vi "crio_RT_Antagonist_Axial_Sine_Sweep.vi"() -> ()   [LabVIEW 2019]
uses:
  <vilib>/LabVIEW Targets/FPGA/cRIO/shared/nicrio_ModuleControls/nicrio_cRIO-9237_ExcitationVoltageRing.ctl
  <vilib>/Platform/TimedLoop/XDataNode/timing_clust.ctl
  <vilib>/Platform/TimedLoop/XDataNode/nitl_modes.ctl
  <vilib>/Platform/TimedLoop/XDataNode/wakeup.ctl
  <vilib>/FPGAPlugInAG/cRIO-9074/niLvFpga_Open_cRIO-9074.vi
  <vilib>/rvi/interface/common/dynamic/niFpgaDynamicAddResources.vi
  <vilib>/Utility/error.llb/Error Cluster From Error Code.vi
  <vilib>/rvi/errors/niLvFpgaAdjustHostInterfaceError.vi
  <vilib>/FPGAPlugInAG/Dynamic/niLvFpga_Close_Dynamic.vi
  <vilib>/rvi/interface/nirviOpenFPGA/nirviOpenFPGA.xnode
  On Call Bitfiles/gpass2_FPGATarget2_crioFPGAAntagoni_YEb8loNiaqg.lvbitx
  <vilib>/rvi/interface/nirviReadWriteControl/nirviReadWriteControl.xnode
  <vilib>/platform/TimedLoop/XDataNode/XDataNode.xnode
  <vilib>/rvi/interface/nirviCloseFPGA/nirviCloseFPGA.xnode
  NiFpgaLv.dll
  <vilib>/rvi/interface/Simulation/niFpgaSimulationCallBeginRW.vi
  <vilib>/Platform/TimedLoop/XDataNode/XDNodeRunTimeDep.lvlib
panel:
  out "PWM":sgl(graph)=0.061072454
  out "Load Cell":dbl(graph)
  in  "LAC Gains":T1={"proportional gain"=0.95454544, "integral gain"=0.64646465} {"proportional gain" scale=0.0..1.0; "integral gain" scale=0.0..1.0}
  in  "LAC Gain Scaler":T1={"proportional gain"=100.0, "integral gain"=100000000.0}
  in  "LAC manual control":T2={"manual? (F)"=FALSE, "manual input (0)"=-0.83838385} {"manual input (0)" scale=-1.0..1.0}
  out "LAC Measured Position":i32
  in  "LAC setpoint":i32(slide) scale=0.0..4500.0
  out "LAC Actual Gain":T1={"proportional gain"=0.009545455, "integral gain"=1.2626262e-09}
  in  "Excitation Voltage":T3 items=["2.5 Volts", "3.3 Volts", "5.0 Volts", "10.0 Volts", "External Excitation"]
  out "Position (Counts) VCA":i32=1
  in  "Lock_debug":bool
  in  "Idle Frequency":dbl=1.0
  in  "Lock_loop_rate":u32=5000
  out "magnitude":fxp<+,32,6>=14.0474853515625
  out "phase (pi)":fxp<+/-,16,2>=0.27923583984375
  out "lock_input":fxp<+/-,16,5>=2.0
  in  "sin_gain":fxp<+,16,2>
  in  "sin_offset":fxp<+/-,16,3>
  out "ControllerPWM Output":sgl=0.5
  out "Mod1/AI0":fxp<+/-,24,-4>=2.2202730178833008e-06
  out "scaled load cell reading":fxp<+/-,24,24>=2.0
  out "Phase":dbl(graph)=-15.1611328125
  out "Phase Graph":cluster{dbl, dbl}[](graph)=[{0.2, -26.400146484375}, {0.25, -26.400146484375}, {0.30000000000000004, -26.982421875}, {0.35000000000000003, -27.70751953125}, {0.4, -27.70751953125}, {0.45, -27.70751953125}, {0.5, -28.80615234375}, {0.55, -28.80615234375}, {0.6000000000000001, -28.80615234375}, {0.65, -29.937744140625}, {0.7, -30.311279296875}, {0.75, -30.311279296875}, {0.8, -31.39892578125}, {0.8500000000000001, -31.915283203125}, {0.9000000000000001, -31.915283203125}, {0.95, -31.915283203125}, {1.0, -32.222900390625}, {1.05, -32.7392578125}, {1.1, -32.84912109375}, {1.1500000000000001, -32.84912109375}, {1.2, -32.84912109375}, {1.25, -33.563232421875}, {1.3, -34.2333984375}, {1.35, -34.2333984375}, {1.4000000000000001, -34.595947265625}, {1.45, -34.947509765625}, {1.5, -35.26611328125}, {1.55, -35.804443359375}, {1.6, -35.804443359375}, {1.6500000000000001, -35.947265625}, {1.7, -36.156005859375}, {1.75, -36.551513671875}, {1.8, -36.595458984375}, {1.85, -36.595458984375}, {1.9000000000000001, -36.93603515625}, {1.95, -36.93603515625}, {2.0, -36.93603515625}, {2.0500000000000003, -37.606201171875}, {2.1, -37.606201171875}, {2.1500000000000004, -38.704833984375}, {2.2, -38.704833984375}, {2.2500000000000004, -38.704833984375}, {2.3000000000000003, -39.3310546875}, {2.35, -39.3310546875}, {2.4000000000000004, -39.3310546875}, {2.45, -40.18798828125}, {2.5000000000000004, -40.18798828125}, {2.5500000000000003, -40.18798828125}, {2.6000000000000005, -41.033935546875}, {2.6500000000000004, -41.033935546875}, {2.7, -41.6162109375}, {2.7500000000000004, -41.6162109375}, {2.8000000000000003, -41.6162109375}, {2.8500000000000005, -42.451171875}, {2.9000000000000004, -42.451171875}, {2.95, -42.91259765625}, {3.0000000000000004, -42.91259765625}, {3.0500000000000003, -42.91259765625}, {3.1000000000000005, -42.91259765625}, {3.1500000000000004, -43.9013671875}, {3.2, -44.9560546875}, {3.2500000000000004, -44.9560546875}, {3.3000000000000003, -44.9560546875}, {3.3500000000000005, -45.46142578125}, {3.4000000000000004, -45.46142578125}, {3.45, -46.680908203125}, {3.5000000000000004, -47.63671875}, {3.5500000000000003, -48.3837890625}, {3.6000000000000005, -48.3837890625}, {3.6500000000000004, -49.339599609375}, {3.7, -49.339599609375}, {3.7500000000000004, -50.372314453125}, {3.8000000000000003, -51.48193359375}, {3.8500000000000005, -51.48193359375}, {3.9000000000000004, -52.283935546875}, {3.95, -52.283935546875}, {4.0, -52.283935546875}, {4.05, -54.60205078125}, {4.1000000000000005, -56.44775390625}, {4.15, -56.44775390625}, {4.2, -57.535400390625}, {4.25, -57.535400390625}, {4.300000000000001, -59.69970703125}, {4.3500000000000005, -62.7978515625}, {4.4, -62.7978515625}, {4.45, -62.7978515625}, {4.5, -66.236572265625}, {4.550000000000001, -66.236572265625}, {4.6000000000000005, -66.236572265625}, {4.65, -66.236572265625}, {4.7, -75.574951171875}, {4.75, -75.574951171875}, {4.800000000000001, -77.838134765625}, {4.8500000000000005, -79.013671875}, {4.9, -79.793701171875}, {4.95, -79.793701171875}, {5.000000000000001, -79.793701171875}, {5.050000000000001, -79.793701171875}, {5.1000000000000005, -86.099853515625}, {5.15, -92.30712890625}, {5.2, -92.30712890625}, {5.250000000000001, -95.8447265625}, {5.300000000000001, -95.8447265625}, {5.3500000000000005, -99.173583984375}, {5.4, -103.831787109375}, {5.45, -103.831787109375}, {5.500000000000001, -105.897216796875}, {5.550000000000001, -105.897216796875}, {5.6000000000000005, -108.6328125}, {5.65, -108.6328125}, {5.7, -108.6328125}, {5.750000000000001, -111.104736328125}, {5.800000000000001, -113.97216796875}, {5.8500000000000005, -113.97216796875}, {5.9, -115.213623046875}, {5.95, -115.213623046875}, {6.000000000000001, -116.0595703125}, {6.050000000000001, -118.092041015625}, {6.1000000000000005, -118.092041015625}, {6.15, -119.190673828125}, {6.2, -120.25634765625}, {6.250000000000001, -120.25634765625}, {6.300000000000001, -122.36572265625}, {6.3500000000000005, -122.607421875}, {6.4, -122.607421875}, {6.45, -123.42041015625}, {6.500000000000001, -123.68408203125}, {6.550000000000001, -123.68408203125}, {6.6000000000000005, -124.420166015625}, {6.65, -124.420166015625}, {6.7, -125.694580078125}, {6.750000000000001, -126.38671875}, {6.800000000000001, -126.375732421875}, {6.8500000000000005, -126.771240234375}, {6.9, -126.771240234375}, {6.95, -127.68310546875}, {7.000000000000001, -128.49609375}, {7.050000000000001, -128.49609375}, {7.1000000000000005, -129.111328125}, {7.15, -129.111328125}, {7.2, -129.111328125}, {7.250000000000001, -129.39697265625}, {7.300000000000001, -130.078125}, {7.3500000000000005, -130.078125}, {7.4, -130.93505859375}, {7.45, -130.93505859375}, {7.500000000000001, -130.93505859375}, {7.550000000000001, -131.85791015625}, {7.6000000000000005, -131.85791015625}, {7.65, -132.42919921875}, {7.7, -132.4951171875}, {7.750000000000001, -132.4951171875}, {7.800000000000001, -134.033203125}, {7.8500000000000005, -134.725341796875}, {7.9, -134.725341796875}, {7.95, -134.912109375}, {8.0, -135.87890625}, {8.05, -136.8017578125}, {8.1, -137.63671875}, {8.15, -137.63671875}, {8.2, -137.63671875}, {8.25, -137.63671875}, {8.299999999999999, -138.5595703125}, {8.35, -138.5595703125}, {8.4, -138.53759765625}, {8.45, -138.53759765625}, {8.5, -138.53759765625}, {8.549999999999999, -138.53759765625}, {8.6, -138.614501953125}, {8.65, -138.614501953125}, {8.7, -138.614501953125}, {8.75, -139.735107421875}, {8.799999999999999, -140.55908203125}, {8.85, -140.55908203125}, {8.9, -141.416015625}, {8.95, -141.778564453125}, {9.0, -141.04248046875}, {9.049999999999999, -141.04248046875}, {9.1, -141.04248046875}, {9.15, -141.4599609375}, {9.2, -141.17431640625}, {9.25, -141.39404296875}, {9.299999999999999, -141.39404296875}, {9.35, -141.48193359375}, {9.4, -142.00927734375}, {9.45, -143.184814453125}, {9.5, -143.536376953125}, {9.549999999999999, -143.536376953125}, {9.6, -143.81103515625}, {9.65, -143.81103515625}, {9.7, -143.81103515625}, {9.75, -143.9208984375}, {9.8, -143.668212890625}, {9.85, -144.173583984375}, {9.9, -144.755859375}, {9.95, -145.316162109375}, {10.0, -145.447998046875}, {10.05, -145.447998046875}, {10.1, -146.173095703125}, {10.15, -146.173095703125}, {10.2, -147.041015625}, {10.25, -146.689453125}, {10.3, -146.689453125}, {10.35, -147.3486328125}, {10.4, -147.3486328125}, {10.45, -148.2275390625}, {10.5, -148.2275390625}, {10.55, -149.710693359375}, {10.6, -149.56787109375}, {10.65, -149.56787109375}, {10.7, -150.347900390625}, {10.75, -150.347900390625}, {10.8, -150.99609375}, {10.85, -150.99609375}, {10.9, -150.99609375}, {10.95, -150.655517578125}, {11.0, -151.380615234375}, {11.05, -151.58935546875}, {11.1, -151.19384765625}, {11.15, -151.8310546875}, {11.2, -151.402587890625}, {11.25, -151.402587890625}, {11.3, -152.138671875}, {11.35, -154.05029296875}, {11.4, -154.05029296875}, {11.45, -155.423583984375}, {11.5, -155.423583984375}, {11.55, -155.379638671875}, {11.6, -154.00634765625}, {11.65, -153.116455078125}, {11.7, -154.039306640625}, {11.75, -154.039306640625}, {11.8, -152.99560546875}, {11.85, -153.555908203125}, {11.9, -153.555908203125}, {11.95, -153.80859375}, {12.0, -153.80859375}, {12.05, -153.80859375}, {12.1, -152.75390625}, {12.15, -154.2919921875}, {12.2, -155.203857421875}, {12.25, -154.281005859375}, {12.3, -153.80859375}, {12.35, -153.80859375}, {12.4, -155.533447265625}, {12.45, -155.533447265625}, {12.5, -155.533447265625}, {12.55, -152.9296875}, {12.6, -152.149658203125}, {12.65, -152.149658203125}, {12.7, -152.55615234375}, {12.75, -152.874755859375}, {12.8, -152.808837890625}, {12.85, -152.720947265625}, {12.9, -152.11669921875}, {12.95, -153.050537109375}, {13.0, -153.204345703125}, {13.05, -154.75341796875}, {13.1, -154.75341796875}, {13.15, -154.852294921875}, {13.2, -152.55615234375}, {13.25, -154.09423828125}, {13.3, -152.2705078125}, {13.35, -152.567138671875}, {13.4, -149.556884765625}, {13.45, -149.974365234375}, {13.5, -153.25927734375}, {13.55, -154.79736328125}, {13.6, -153.863525390625}, {13.65, -155.32470703125}, {13.7, -155.3466796875}, {13.75, -155.21484375}, {13.8, -155.54443359375}, {13.85, -156.15966796875}, {13.9, -156.15966796875}, {13.95, -157.115478515625}, {14.0, -157.1484375}, {14.05, -157.7197265625}, {14.1, -157.774658203125}, {14.15, -157.774658203125}, {14.2, -157.774658203125}, {14.25, -157.774658203125}, {14.3, -157.74169921875}, {14.35, -157.74169921875}, {14.4, -157.74169921875}, {14.45, -158.104248046875}, {14.5, -158.0712890625}, {14.55, -158.09326171875}, {14.6, -158.09326171875}, {14.65, -158.09326171875}, {14.7, -157.587890625}, {14.75, -157.74169921875}, {14.8, -157.74169921875}, {14.85, -157.379150390625}, {14.9, -157.03857421875}, {14.95, -157.03857421875}, {15.0, -157.554931640625}, {15.05, -158.22509765625}, {15.1, -157.928466796875}, {15.15, -157.928466796875}, {15.2, -158.26904296875}, {15.25, -158.26904296875}, {15.3, -158.082275390625}, {15.35, -158.082275390625}, {15.4, -157.412109375}, {15.45, -156.851806640625}, {15.5, -156.851806640625}, {15.55, -158.2470703125}, {15.6, -157.598876953125}, {15.65, -158.060302734375}, {15.7, -158.060302734375}, {15.75, -157.9833984375}, {15.8, -158.18115234375}, {15.85, -158.2470703125}, {15.9, -158.016357421875}, {15.95, -158.88427734375}, {16.0, -158.88427734375}, {16.05, -158.66455078125}, {16.1, -158.66455078125}, {16.150000000000002, -158.62060546875}, {16.2, -158.62060546875}, {16.25, -158.236083984375}, {16.3, -158.70849609375}, {16.35, -159.06005859375}, {16.4, -159.06005859375}, {16.45, -160.147705078125}, {16.5, -160.147705078125}, {16.55, -159.598388671875}, {16.6, -159.3017578125}, {16.65, -159.378662109375}, {16.7, -159.609375}, {16.75, -158.40087890625}, {16.8, -158.40087890625}, {16.85, -160.33447265625}, {16.9, -159.98291015625}, {16.95, -159.598388671875}, {17.0, -159.54345703125}, {17.05, -159.54345703125}, {17.1, -157.91748046875}, {17.15, -157.91748046875}, {17.2, -159.027099609375}, {17.25, -160.279541015625}, {17.3, -160.279541015625}, {17.35, -158.79638671875}, {17.4, -158.038330078125}, {17.45, -158.038330078125}, {17.5, -158.5986328125}, {17.55, -160.147705078125}, {17.6, -158.62060546875}, {17.65, -157.840576171875}, {17.7, -157.840576171875}, {17.75, -157.840576171875}, {17.8, -157.840576171875}, {17.85, -158.675537109375}, {17.9, -160.279541015625}, {17.95, -158.280029296875}, {18.0, -157.686767578125}, {18.05, -157.686767578125}, {18.1, -157.115478515625}, {18.15, -157.236328125}, {18.2, -157.027587890625}, {18.25, -158.00537109375}, {18.3, -158.00537109375}, {18.35, -158.00537109375}, {18.4, -156.4892578125}, {18.45, -157.093505859375}, {18.5, -159.246826171875}, {18.55, -159.10400390625}, {18.6, -159.41162109375}, {18.65, -159.0380859375}, {18.7, -158.31298828125}, {18.75, -160.257568359375}, {18.8, -160.48828125}, {18.85, -159.971923828125}, {18.9, -159.63134765625}, {18.95, -159.63134765625}, {19.0, -159.63134765625}, {19.05, -158.994140625}, {19.1, -159.686279296875}, {19.15, -161.455078125}, {19.2, -161.3671875}, {19.25, -160.806884765625}, {19.3, -160.806884765625}, {19.35, -159.58740234375}, {19.400000000000002, -162.13623046875}, {19.45, -161.795654296875}, {19.5, -161.19140625}, {19.55, -161.19140625}, {19.6, -161.19140625}, {19.650000000000002, -161.19140625}, {19.7, -160.224609375}, {19.75, -160.224609375}, {19.8, -159.444580078125}, {19.85, -161.279296875}, {19.900000000000002, -161.5869140625}, {19.95, -161.38916015625}, {20.0, -160.675048828125}, {20.05, -159.76318359375}, {20.1, -51.6357421875}, {20.150000000000002, -15.1611328125}]
  out "Magnitude":dbl(graph)=2.4527311325073242e-05
  out "Amplitude Graph":cluster{dbl, dbl}[](graph)=[{0.2, 0.03331726789474487}, {0.25, 0.03331726789474487}, {0.30000000000000004, 0.10618984699249268}, {0.35000000000000003, 0.10533280670642853}, {0.4, 0.10533280670642853}, {0.45, 0.10533280670642853}, {0.5, 0.1050892174243927}, {0.55, 0.1050892174243927}, {0.6000000000000001, 0.1050892174243927}, {0.65, 0.1055905669927597}, {0.7, 0.1055905669927597}, {0.75, 0.10717682540416718}, {0.8, 0.10736270248889923}, {0.8500000000000001, 0.10746829211711884}, {0.9000000000000001, 0.10746829211711884}, {0.95, 0.10746829211711884}, {1.0, 0.1083083301782608}, {1.05, 0.10839883983135223}, {1.1, 0.10935868322849274}, {1.1500000000000001, 0.10935868322849274}, {1.2, 0.10935868322849274}, {1.25, 0.1103353351354599}, {1.3, 0.11236743628978729}, {1.35, 0.11236743628978729}, {1.4000000000000001, 0.11426505446434021}, {1.45, 0.11589774489402771}, {1.5, 0.11667266488075256}, {1.55, 0.11638469994068146}, {1.6, 0.11638469994068146}, {1.6500000000000001, 0.11864681541919708}, {1.7, 0.11830170452594757}, {1.75, 0.11777929961681366}, {1.8, 0.11881615221500397}, {1.85, 0.11881615221500397}, {1.9000000000000001, 0.11973647773265839}, {1.95, 0.11973647773265839}, {2.0, 0.11973647773265839}, {2.0500000000000003, 0.1216040849685669}, {2.1, 0.1216040849685669}, {2.1500000000000004, 0.12410874664783478}, {2.2, 0.12410874664783478}, {2.2500000000000004, 0.12410874664783478}, {2.3000000000000003, 0.12537233531475067}, {2.35, 0.12537233531475067}, {2.4000000000000004, 0.12537233531475067}, {2.45, 0.1261354684829712}, {2.5000000000000004, 0.1261354684829712}, {2.5500000000000003, 0.1261354684829712}, {2.6000000000000005, 0.12728527188301086}, {2.6500000000000004, 0.12728527188301086}, {2.7, 0.1275573968887329}, {2.7500000000000004, 0.1275573968887329}, {2.8000000000000003, 0.1275573968887329}, {2.8500000000000005, 0.13189205527305603}, {2.9000000000000004, 0.13189205527305603}, {2.95, 0.13356561958789825}, {3.0000000000000004, 0.13356561958789825}, {3.0500000000000003, 0.13356561958789825}, {3.1000000000000005, 0.13356561958789825}, {3.1500000000000004, 0.13717493414878845}, {3.2, 0.14104332029819489}, {3.2500000000000004, 0.14104332029819489}, {3.3000000000000003, 0.14104332029819489}, {3.3500000000000005, 0.14525270462036133}, {3.4000000000000004, 0.14525270462036133}, {3.45, 0.14957602322101593}, {3.5000000000000004, 0.15649737417697906}, {3.5500000000000003, 0.15769919753074646}, {3.6000000000000005, 0.15769919753074646}, {3.6500000000000004, 0.16097605228424072}, {3.7, 0.16097605228424072}, {3.7500000000000004, 0.1667061746120453}, {3.8000000000000003, 0.1725185215473175}, {3.8500000000000005, 0.1725185215473175}, {3.9000000000000004, 0.17658789455890656}, {3.95, 0.17658789455890656}, {4.0, 0.17658789455890656}, {4.05, 0.18601292371749878}, {4.1000000000000005, 0.1940435916185379}, {4.15, 0.1940435916185379}, {4.2, 0.198423832654953}, {4.25, 0.198423832654953}, {4.300000000000001, 0.2107202559709549}, {4.3500000000000005, 0.22146329283714294}, {4.4, 0.22146329283714294}, {4.45, 0.22146329283714294}, {4.5, 0.235212042927742}, {4.550000000000001, 0.235212042927742}, {4.6000000000000005, 0.235212042927742}, {4.65, 0.235212042927742}, {4.7, 0.2640381157398224}, {4.75, 0.2640381157398224}, {4.800000000000001, 0.26513098180294037}, {4.8500000000000005, 0.26586630940437317}, {4.9, 0.2656572312116623}, {4.95, 0.2656572312116623}, {5.000000000000001, 0.2656572312116623}, {5.050000000000001, 0.2656572312116623}, {5.1000000000000005, 0.26507458090782166}, {5.15, 0.2656416743993759}, {5.2, 0.2656416743993759}, {5.250000000000001, 0.251346692442894}, {5.300000000000001, 0.251346692442894}, {5.3500000000000005, 0.2536720186471939}, {5.4, 0.2437794953584671}, {5.45, 0.2437794953584671}, {5.500000000000001, 0.23735088109970093}, {5.550000000000001, 0.23735088109970093}, {5.6000000000000005, 0.22691191732883453}, {5.65, 0.22691191732883453}, {5.7, 0.22691191732883453}, {5.750000000000001, 0.21705244481563568}, {5.800000000000001, 0.20304445922374725}, {5.8500000000000005, 0.20304445922374725}, {5.9, 0.19810320436954498}, {5.95, 0.19810320436954498}, {6.000000000000001, 0.18994279205799103}, {6.050000000000001, 0.17516598105430603}, {6.1000000000000005, 0.17516598105430603}, {6.15, 0.17183275520801544}, {6.2, 0.1663980633020401}, {6.250000000000001, 0.1663980633020401}, {6.300000000000001, 0.16198883950710297}, {6.3500000000000005, 0.149206280708313}, {6.4, 0.149206280708313}, {6.45, 0.1458333134651184}, {6.500000000000001, 0.14127014577388763}, {6.550000000000001, 0.14127014577388763}, {6.6000000000000005, 0.1334792673587799}, {6.65, 0.1334792673587799}, {6.7, 0.1280384361743927}, {6.750000000000001, 0.12309364974498749}, {6.800000000000001, 0.12037937343120575}, {6.8500000000000005, 0.11749586462974548}, {6.9, 0.11749586462974548}, {6.95, 0.1133015900850296}, {7.000000000000001, 0.1110016256570816}, {7.050000000000001, 0.1110016256570816}, {7.1000000000000005, 0.10756750404834747}, {7.15, 0.10756750404834747}, {7.2, 0.10756750404834747}, {7.250000000000001, 0.10231640934944153}, {7.300000000000001, 0.09651859104633331}, {7.3500000000000005, 0.09651859104633331}, {7.4, 0.09285260736942291}, {7.45, 0.09285260736942291}, {7.500000000000001, 0.09285260736942291}, {7.550000000000001, 0.09010781347751617}, {7.6000000000000005, 0.09010781347751617}, {7.65, 0.08745460212230682}, {7.7, 0.08326256275177002}, {7.750000000000001, 0.08326256275177002}, {7.800000000000001, 0.08057750761508942}, {7.8500000000000005, 0.07818682491779327}, {7.9, 0.07818682491779327}, {7.95, 0.07696442306041718}, {8.0, 0.07506111264228821}, {8.05, 0.07425171136856079}, {8.1, 0.07347100973129272}, {8.15, 0.07347100973129272}, {8.2, 0.07347100973129272}, {8.25, 0.07347100973129272}, {8.299999999999999, 0.07046669721603394}, {8.35, 0.07046669721603394}, {8.4, 0.06673818826675415}, {8.45, 0.06673818826675415}, {8.5, 0.06673818826675415}, {8.549999999999999, 0.06673818826675415}, {8.6, 0.06287001073360443}, {8.65, 0.06287001073360443}, {8.7, 0.06287001073360443}, {8.75, 0.06020982563495636}, {8.799999999999999, 0.059322893619537354}, {8.85, 0.059322893619537354}, {8.9, 0.05871616303920746}, {8.95, 0.057818397879600525}, {9.0, 0.05670835077762604}, {9.049999999999999, 0.05670835077762604}, {9.1, 0.05670835077762604}, {9.15, 0.0519668310880661}, {9.2, 0.04866628348827362}, {9.25, 0.04656481742858887}, {9.299999999999999, 0.04656481742858887}, {9.35, 0.045131951570510864}, {9.4, 0.044366300106048584}, {9.45, 0.04485899209976196}, {9.5, 0.04394112527370453}, {9.549999999999999, 0.04394112527370453}, {9.6, 0.04320792853832245}, {9.65, 0.04320792853832245}, {9.7, 0.04320792853832245}, {9.75, 0.0410747230052948}, {9.8, 0.039193376898765564}, {9.85, 0.039149269461631775}, {9.9, 0.03955969214439392}, {9.95, 0.03950272500514984}, {10.0, 0.03950531780719757}, {10.05, 0.03950531780719757}, {10.1, 0.038819193840026855}, {10.15, 0.038819193840026855}, {10.2, 0.03834253549575806}, {10.25, 0.03784604370594025}, {10.3, 0.03784604370594025}, {10.35, 0.037662506103515625}, {10.4, 0.037662506103515625}, {10.45, 0.03731667995452881}, {10.5, 0.03731667995452881}, {10.55, 0.03716094791889191}, {10.6, 0.036722585558891296}, {10.65, 0.036722585558891296}, {10.7, 0.03586658835411072}, {10.75, 0.03586658835411072}, {10.8, 0.03571528196334839}, {10.85, 0.03571528196334839}, {10.9, 0.03571528196334839}, {10.95, 0.035297706723213196}, {11.0, 0.03483690321445465}, {11.05, 0.03411737084388733}, {11.1, 0.034097686409950256}, {11.15, 0.03402881324291229}, {11.2, 0.03402455151081085}, {11.25, 0.03402455151081085}, {11.3, 0.03317683935165405}, {11.35, 0.03293997049331665}, {11.4, 0.03293997049331665}, {11.45, 0.032306089997291565}, {11.5, 0.032306089997291565}, {11.55, 0.03184396028518677}, {11.6, 0.03126631677150726}, {11.65, 0.03090965747833252}, {11.7, 0.03021879494190216}, {11.75, 0.03021879494190216}, {11.8, 0.030169516801834106}, {11.85, 0.029628857970237732}, {11.9, 0.029628857970237732}, {11.95, 0.029396548867225647}, {12.0, 0.029396548867225647}, {12.05, 0.029396548867225647}, {12.1, 0.02890034019947052}, {12.15, 0.02848656475543976}, {12.2, 0.028094440698623657}, {12.25, 0.027950122952461243}, {12.3, 0.027714908123016357}, {12.35, 0.027714908123016357}, {12.4, 0.02662232518196106}, {12.45, 0.02662232518196106}, {12.5, 0.02662232518196106}, {12.55, 0.02711588144302368}, {12.6, 0.026656121015548706}, {12.65, 0.026656121015548706}, {12.7, 0.02646125853061676}, {12.75, 0.02592301368713379}, {12.8, 0.026159614324569702}, {12.85, 0.026123300194740295}, {12.9, 0.025856971740722656}, {12.95, 0.025539815425872803}, {13.0, 0.025329887866973877}, {13.05, 0.02516321837902069}, {13.1, 0.02516321837902069}, {13.15, 0.024456799030303955}, {13.2, 0.024328216910362244}, {13.25, 0.023910611867904663}, {13.3, 0.023622646927833557}, {13.35, 0.02343292534351349}, {13.4, 0.02223210036754608}, {13.45, 0.020938292145729065}, {13.5, 0.020729809999465942}, {13.55, 0.020074576139450073}, {13.6, 0.019756391644477844}, {13.65, 0.019418329000473022}, {13.7, 0.019466668367385864}, {13.75, 0.019271820783615112}, {13.8, 0.018854692578315735}, {13.85, 0.01883484423160553}, {13.9, 0.01883484423160553}, {13.95, 0.018730804324150085}, {14.0, 0.018973082304000854}, {14.05, 0.018952399492263794}, {14.1, 0.01899656653404236}, {14.15, 0.01899656653404236}, {14.2, 0.01899656653404236}, {14.25, 0.01899656653404236}, {14.3, 0.018805980682373047}, {14.35, 0.018805980682373047}, {14.4, 0.018805980682373047}, {14.45, 0.018020927906036377}, {14.5, 0.017717868089675903}, {14.55, 0.017765402793884277}, {14.6, 0.017765402793884277}, {14.65, 0.017765402793884277}, {14.7, 0.017564281821250916}, {14.75, 0.017058134078979492}, {14.8, 0.017058134078979492}, {14.85, 0.016754895448684692}, {14.9, 0.01626691222190857}, {14.95, 0.01626691222190857}, {15.0, 0.015460893511772156}, {15.05, 0.01572345197200775}, {15.1, 0.01582910120487213}, {15.15, 0.01582910120487213}, {15.2, 0.015757665038108826}, {15.25, 0.015757665038108826}, {15.3, 0.015610411763191223}, {15.35, 0.015610411763191223}, {15.4, 0.015372350811958313}, {15.45, 0.015085607767105103}, {15.5, 0.015085607767105103}, {15.55, 0.015382200479507446}, {15.6, 0.015127897262573242}, {15.65, 0.015146493911743164}, {15.7, 0.015146493911743164}, {15.75, 0.015044525265693665}, {15.8, 0.01474955677986145}, {15.85, 0.014485776424407959}, {15.9, 0.014271214604377747}, {15.95, 0.014475688338279724}, {16.0, 0.014475688338279724}, {16.05, 0.014406517148017883}, {16.1, 0.014406517148017883}, {16.150000000000002, 0.013971179723739624}, {16.2, 0.013971179723739624}, {16.25, 0.013821527361869812}, {16.3, 0.0132923424243927}, {16.35, 0.013130217790603638}, {16.4, 0.013130217790603638}, {16.45, 0.012945547699928284}, {16.5, 0.012945547699928284}, {16.55, 0.012944266200065613}, {16.6, 0.012709051370620728}, {16.65, 0.012769058346748352}, {16.7, 0.012716874480247498}, {16.75, 0.012297123670578003}, {16.8, 0.012297123670578003}, {16.85, 0.012073531746864319}, {16.9, 0.012110486626625061}, {16.95, 0.012085676193237305}, {17.0, 0.012085676193237305}, {17.05, 0.01193799078464508}, {17.1, 0.011186644434928894}, {17.15, 0.011186644434928894}, {17.2, 0.01080833375453949}, {17.25, 0.010843172669410706}, {17.3, 0.010843172669410706}, {17.35, 0.010700181126594543}, {17.4, 0.010160878300666809}, {17.45, 0.010160878300666809}, {17.5, 0.009855195879936218}, {17.55, 0.009873896837234497}, {17.6, 0.009833112359046936}, {17.65, 0.00976167619228363}, {17.7, 0.00976167619228363}, {17.75, 0.00976167619228363}, {17.8, 0.009272292256355286}, {17.85, 0.009257376194000244}, {17.9, 0.009209305047988892}, {17.95, 0.00928729772567749}, {18.0, 0.008991464972496033}, {18.05, 0.008991464972496033}, {18.1, 0.008727356791496277}, {18.15, 0.008638560771942139}, {18.2, 0.008453026413917542}, {18.25, 0.008413761854171753}, {18.3, 0.008413761854171753}, {18.35, 0.008413761854171753}, {18.4, 0.007322326302528381}, {18.45, 0.007352367043495178}, {18.5, 0.008893147110939026}, {18.55, 0.008593544363975525}, {18.6, 0.008684352040290833}, {18.65, 0.00877903401851654}, {18.7, 0.008505448698997498}, {18.75, 0.008388862013816833}, {18.8, 0.008554816246032715}, {18.85, 0.008490398526191711}, {18.9, 0.008520618081092834}, {18.95, 0.008520618081092834}, {19.0, 0.008520618081092834}, {19.05, 0.008324384689331055}, {19.1, 0.007978126406669617}, {19.15, 0.007994204759597778}, {19.2, 0.008034005761146545}, {19.25, 0.007959425449371338}, {19.3, 0.007959425449371338}, {19.35, 0.00761200487613678}, {19.400000000000002, 0.007574364542961121}, {19.45, 0.007543906569480896}, {19.5, 0.007398888468742371}, {19.55, 0.007398888468742371}, {19.6, 0.007398888468742371}, {19.650000000000002, 0.007398888468742371}, {19.7, 0.007126152515411377}, {19.75, 0.007126152515411377}, {19.8, 0.0067656636238098145}, {19.85, 0.0066679418087005615}, {19.900000000000002, 0.006978675723075867}, {19.95, 0.006995022296905518}, {20.0, 0.006885826587677002}, {20.05, 0.006692931056022644}, {20.1, 3.5822391510009766e-05}, {20.150000000000002, 2.4527311325073242e-05}]
  out "Absolute Force":dbl(graph)=2.4527311325073242e-05
  out "Absolute Amplitude":cluster{dbl, dbl}[](graph)=[{0.2, 0.03331726789474487}, {0.25, 0.03331726789474487}, {0.30000000000000004, 0.10618984699249268}, {0.35000000000000003, 0.10533280670642853}, {0.4, 0.10533280670642853}, {0.45, 0.10533280670642853}, {0.5, 0.1050892174243927}, {0.55, 0.1050892174243927}, {0.6000000000000001, 0.1050892174243927}, {0.65, 0.1055905669927597}, {0.7, 0.1055905669927597}, {0.75, 0.10717682540416718}, {0.8, 0.10736270248889923}, {0.8500000000000001, 0.10746829211711884}, {0.9000000000000001, 0.10746829211711884}, {0.95, 0.10746829211711884}, {1.0, 0.1083083301782608}, {1.05, 0.10839883983135223}, {1.1, 0.10935868322849274}, {1.1500000000000001, 0.10935868322849274}, {1.2, 0.10935868322849274}, {1.25, 0.1103353351354599}, {1.3, 0.11236743628978729}, {1.35, 0.11236743628978729}, {1.4000000000000001, 0.11426505446434021}, {1.45, 0.11589774489402771}, {1.5, 0.11667266488075256}, {1.55, 0.11638469994068146}, {1.6, 0.11638469994068146}, {1.6500000000000001, 0.11864681541919708}, {1.7, 0.11830170452594757}, {1.75, 0.11777929961681366}, {1.8, 0.11881615221500397}, {1.85, 0.11881615221500397}, {1.9000000000000001, 0.11973647773265839}, {1.95, 0.11973647773265839}, {2.0, 0.11973647773265839}, {2.0500000000000003, 0.1216040849685669}, {2.1, 0.1216040849685669}, {2.1500000000000004, 0.12410874664783478}, {2.2, 0.12410874664783478}, {2.2500000000000004, 0.12410874664783478}, {2.3000000000000003, 0.12537233531475067}, {2.35, 0.12537233531475067}, {2.4000000000000004, 0.12537233531475067}, {2.45, 0.1261354684829712}, {2.5000000000000004, 0.1261354684829712}, {2.5500000000000003, 0.1261354684829712}, {2.6000000000000005, 0.12728527188301086}, {2.6500000000000004, 0.12728527188301086}, {2.7, 0.1275573968887329}, {2.7500000000000004, 0.1275573968887329}, {2.8000000000000003, 0.1275573968887329}, {2.8500000000000005, 0.13189205527305603}, {2.9000000000000004, 0.13189205527305603}, {2.95, 0.13356561958789825}, {3.0000000000000004, 0.13356561958789825}, {3.0500000000000003, 0.13356561958789825}, {3.1000000000000005, 0.13356561958789825}, {3.1500000000000004, 0.13717493414878845}, {3.2, 0.14104332029819489}, {3.2500000000000004, 0.14104332029819489}, {3.3000000000000003, 0.14104332029819489}, {3.3500000000000005, 0.14525270462036133}, {3.4000000000000004, 0.14525270462036133}, {3.45, 0.14957602322101593}, {3.5000000000000004, 0.15649737417697906}, {3.5500000000000003, 0.15769919753074646}, {3.6000000000000005, 0.15769919753074646}, {3.6500000000000004, 0.16097605228424072}, {3.7, 0.16097605228424072}, {3.7500000000000004, 0.1667061746120453}, {3.8000000000000003, 0.1725185215473175}, {3.8500000000000005, 0.1725185215473175}, {3.9000000000000004, 0.17658789455890656}, {3.95, 0.17658789455890656}, {4.0, 0.17658789455890656}, {4.05, 0.18601292371749878}, {4.1000000000000005, 0.1940435916185379}, {4.15, 0.1940435916185379}, {4.2, 0.198423832654953}, {4.25, 0.198423832654953}, {4.300000000000001, 0.2107202559709549}, {4.3500000000000005, 0.22146329283714294}, {4.4, 0.22146329283714294}, {4.45, 0.22146329283714294}, {4.5, 0.235212042927742}, {4.550000000000001, 0.235212042927742}, {4.6000000000000005, 0.235212042927742}, {4.65, 0.235212042927742}, {4.7, 0.2640381157398224}, {4.75, 0.2640381157398224}, {4.800000000000001, 0.26513098180294037}, {4.8500000000000005, 0.26586630940437317}, {4.9, 0.2656572312116623}, {4.95, 0.2656572312116623}, {5.000000000000001, 0.2656572312116623}, {5.050000000000001, 0.2656572312116623}, {5.1000000000000005, 0.26507458090782166}, {5.15, 0.2656416743993759}, {5.2, 0.2656416743993759}, {5.250000000000001, 0.251346692442894}, {5.300000000000001, 0.251346692442894}, {5.3500000000000005, 0.2536720186471939}, {5.4, 0.2437794953584671}, {5.45, 0.2437794953584671}, {5.500000000000001, 0.23735088109970093}, {5.550000000000001, 0.23735088109970093}, {5.6000000000000005, 0.22691191732883453}, {5.65, 0.22691191732883453}, {5.7, 0.22691191732883453}, {5.750000000000001, 0.21705244481563568}, {5.800000000000001, 0.20304445922374725}, {5.8500000000000005, 0.20304445922374725}, {5.9, 0.19810320436954498}, {5.95, 0.19810320436954498}, {6.000000000000001, 0.18994279205799103}, {6.050000000000001, 0.17516598105430603}, {6.1000000000000005, 0.17516598105430603}, {6.15, 0.17183275520801544}, {6.2, 0.1663980633020401}, {6.250000000000001, 0.1663980633020401}, {6.300000000000001, 0.16198883950710297}, {6.3500000000000005, 0.149206280708313}, {6.4, 0.149206280708313}, {6.45, 0.1458333134651184}, {6.500000000000001, 0.14127014577388763}, {6.550000000000001, 0.14127014577388763}, {6.6000000000000005, 0.1334792673587799}, {6.65, 0.1334792673587799}, {6.7, 0.1280384361743927}, {6.750000000000001, 0.12309364974498749}, {6.800000000000001, 0.12037937343120575}, {6.8500000000000005, 0.11749586462974548}, {6.9, 0.11749586462974548}, {6.95, 0.1133015900850296}, {7.000000000000001, 0.1110016256570816}, {7.050000000000001, 0.1110016256570816}, {7.1000000000000005, 0.10756750404834747}, {7.15, 0.10756750404834747}, {7.2, 0.10756750404834747}, {7.250000000000001, 0.10231640934944153}, {7.300000000000001, 0.09651859104633331}, {7.3500000000000005, 0.09651859104633331}, {7.4, 0.09285260736942291}, {7.45, 0.09285260736942291}, {7.500000000000001, 0.09285260736942291}, {7.550000000000001, 0.09010781347751617}, {7.6000000000000005, 0.09010781347751617}, {7.65, 0.08745460212230682}, {7.7, 0.08326256275177002}, {7.750000000000001, 0.08326256275177002}, {7.800000000000001, 0.08057750761508942}, {7.8500000000000005, 0.07818682491779327}, {7.9, 0.07818682491779327}, {7.95, 0.07696442306041718}, {8.0, 0.07506111264228821}, {8.05, 0.07425171136856079}, {8.1, 0.07347100973129272}, {8.15, 0.07347100973129272}, {8.2, 0.07347100973129272}, {8.25, 0.07347100973129272}, {8.299999999999999, 0.07046669721603394}, {8.35, 0.07046669721603394}, {8.4, 0.06673818826675415}, {8.45, 0.06673818826675415}, {8.5, 0.06673818826675415}, {8.549999999999999, 0.06673818826675415}, {8.6, 0.06287001073360443}, {8.65, 0.06287001073360443}, {8.7, 0.06287001073360443}, {8.75, 0.06020982563495636}, {8.799999999999999, 0.059322893619537354}, {8.85, 0.059322893619537354}, {8.9, 0.05871616303920746}, {8.95, 0.057818397879600525}, {9.0, 0.05670835077762604}, {9.049999999999999, 0.05670835077762604}, {9.1, 0.05670835077762604}, {9.15, 0.0519668310880661}, {9.2, 0.04866628348827362}, {9.25, 0.04656481742858887}, {9.299999999999999, 0.04656481742858887}, {9.35, 0.045131951570510864}, {9.4, 0.044366300106048584}, {9.45, 0.04485899209976196}, {9.5, 0.04394112527370453}, {9.549999999999999, 0.04394112527370453}, {9.6, 0.04320792853832245}, {9.65, 0.04320792853832245}, {9.7, 0.04320792853832245}, {9.75, 0.0410747230052948}, {9.8, 0.039193376898765564}, {9.85, 0.039149269461631775}, {9.9, 0.03955969214439392}, {9.95, 0.03950272500514984}, {10.0, 0.03950531780719757}, {10.05, 0.03950531780719757}, {10.1, 0.038819193840026855}, {10.15, 0.038819193840026855}, {10.2, 0.03834253549575806}, {10.25, 0.03784604370594025}, {10.3, 0.03784604370594025}, {10.35, 0.037662506103515625}, {10.4, 0.037662506103515625}, {10.45, 0.03731667995452881}, {10.5, 0.03731667995452881}, {10.55, 0.03716094791889191}, {10.6, 0.036722585558891296}, {10.65, 0.036722585558891296}, {10.7, 0.03586658835411072}, {10.75, 0.03586658835411072}, {10.8, 0.03571528196334839}, {10.85, 0.03571528196334839}, {10.9, 0.03571528196334839}, {10.95, 0.035297706723213196}, {11.0, 0.03483690321445465}, {11.05, 0.03411737084388733}, {11.1, 0.034097686409950256}, {11.15, 0.03402881324291229}, {11.2, 0.03402455151081085}, {11.25, 0.03402455151081085}, {11.3, 0.03317683935165405}, {11.35, 0.03293997049331665}, {11.4, 0.03293997049331665}, {11.45, 0.032306089997291565}, {11.5, 0.032306089997291565}, {11.55, 0.03184396028518677}, {11.6, 0.03126631677150726}, {11.65, 0.03090965747833252}, {11.7, 0.03021879494190216}, {11.75, 0.03021879494190216}, {11.8, 0.030169516801834106}, {11.85, 0.029628857970237732}, {11.9, 0.029628857970237732}, {11.95, 0.029396548867225647}, {12.0, 0.029396548867225647}, {12.05, 0.029396548867225647}, {12.1, 0.02890034019947052}, {12.15, 0.02848656475543976}, {12.2, 0.028094440698623657}, {12.25, 0.027950122952461243}, {12.3, 0.027714908123016357}, {12.35, 0.027714908123016357}, {12.4, 0.02662232518196106}, {12.45, 0.02662232518196106}, {12.5, 0.02662232518196106}, {12.55, 0.02711588144302368}, {12.6, 0.026656121015548706}, {12.65, 0.026656121015548706}, {12.7, 0.02646125853061676}, {12.75, 0.02592301368713379}, {12.8, 0.026159614324569702}, {12.85, 0.026123300194740295}, {12.9, 0.025856971740722656}, {12.95, 0.025539815425872803}, {13.0, 0.025329887866973877}, {13.05, 0.02516321837902069}, {13.1, 0.02516321837902069}, {13.15, 0.024456799030303955}, {13.2, 0.024328216910362244}, {13.25, 0.023910611867904663}, {13.3, 0.023622646927833557}, {13.35, 0.02343292534351349}, {13.4, 0.02223210036754608}, {13.45, 0.020938292145729065}, {13.5, 0.020729809999465942}, {13.55, 0.020074576139450073}, {13.6, 0.019756391644477844}, {13.65, 0.019418329000473022}, {13.7, 0.019466668367385864}, {13.75, 0.019271820783615112}, {13.8, 0.018854692578315735}, {13.85, 0.01883484423160553}, {13.9, 0.01883484423160553}, {13.95, 0.018730804324150085}, {14.0, 0.018973082304000854}, {14.05, 0.018952399492263794}, {14.1, 0.01899656653404236}, {14.15, 0.01899656653404236}, {14.2, 0.01899656653404236}, {14.25, 0.01899656653404236}, {14.3, 0.018805980682373047}, {14.35, 0.018805980682373047}, {14.4, 0.018805980682373047}, {14.45, 0.018020927906036377}, {14.5, 0.017717868089675903}, {14.55, 0.017765402793884277}, {14.6, 0.017765402793884277}, {14.65, 0.017765402793884277}, {14.7, 0.017564281821250916}, {14.75, 0.017058134078979492}, {14.8, 0.017058134078979492}, {14.85, 0.016754895448684692}, {14.9, 0.01626691222190857}, {14.95, 0.01626691222190857}, {15.0, 0.015460893511772156}, {15.05, 0.01572345197200775}, {15.1, 0.01582910120487213}, {15.15, 0.01582910120487213}, {15.2, 0.015757665038108826}, {15.25, 0.015757665038108826}, {15.3, 0.015610411763191223}, {15.35, 0.015610411763191223}, {15.4, 0.015372350811958313}, {15.45, 0.015085607767105103}, {15.5, 0.015085607767105103}, {15.55, 0.015382200479507446}, {15.6, 0.015127897262573242}, {15.65, 0.015146493911743164}, {15.7, 0.015146493911743164}, {15.75, 0.015044525265693665}, {15.8, 0.01474955677986145}, {15.85, 0.014485776424407959}, {15.9, 0.014271214604377747}, {15.95, 0.014475688338279724}, {16.0, 0.014475688338279724}, {16.05, 0.014406517148017883}, {16.1, 0.014406517148017883}, {16.150000000000002, 0.013971179723739624}, {16.2, 0.013971179723739624}, {16.25, 0.013821527361869812}, {16.3, 0.0132923424243927}, {16.35, 0.013130217790603638}, {16.4, 0.013130217790603638}, {16.45, 0.012945547699928284}, {16.5, 0.012945547699928284}, {16.55, 0.012944266200065613}, {16.6, 0.012709051370620728}, {16.65, 0.012769058346748352}, {16.7, 0.012716874480247498}, {16.75, 0.012297123670578003}, {16.8, 0.012297123670578003}, {16.85, 0.012073531746864319}, {16.9, 0.012110486626625061}, {16.95, 0.012085676193237305}, {17.0, 0.012085676193237305}, {17.05, 0.01193799078464508}, {17.1, 0.011186644434928894}, {17.15, 0.011186644434928894}, {17.2, 0.01080833375453949}, {17.25, 0.010843172669410706}, {17.3, 0.010843172669410706}, {17.35, 0.010700181126594543}, {17.4, 0.010160878300666809}, {17.45, 0.010160878300666809}, {17.5, 0.009855195879936218}, {17.55, 0.009873896837234497}, {17.6, 0.009833112359046936}, {17.65, 0.00976167619228363}, {17.7, 0.00976167619228363}, {17.75, 0.00976167619228363}, {17.8, 0.009272292256355286}, {17.85, 0.009257376194000244}, {17.9, 0.009209305047988892}, {17.95, 0.00928729772567749}, {18.0, 0.008991464972496033}, {18.05, 0.008991464972496033}, {18.1, 0.008727356791496277}, {18.15, 0.008638560771942139}, {18.2, 0.008453026413917542}, {18.25, 0.008413761854171753}, {18.3, 0.008413761854171753}, {18.35, 0.008413761854171753}, {18.4, 0.007322326302528381}, {18.45, 0.007352367043495178}, {18.5, 0.008893147110939026}, {18.55, 0.008593544363975525}, {18.6, 0.008684352040290833}, {18.65, 0.00877903401851654}, {18.7, 0.008505448698997498}, {18.75, 0.008388862013816833}, {18.8, 0.008554816246032715}, {18.85, 0.008490398526191711}, {18.9, 0.008520618081092834}, {18.95, 0.008520618081092834}, {19.0, 0.008520618081092834}, {19.05, 0.008324384689331055}, {19.1, 0.007978126406669617}, {19.15, 0.007994204759597778}, {19.2, 0.008034005761146545}, {19.25, 0.007959425449371338}, {19.3, 0.007959425449371338}, {19.35, 0.00761200487613678}, {19.400000000000002, 0.007574364542961121}, {19.45, 0.007543906569480896}, {19.5, 0.007398888468742371}, {19.55, 0.007398888468742371}, {19.6, 0.007398888468742371}, {19.650000000000002, 0.007398888468742371}, {19.7, 0.007126152515411377}, {19.75, 0.007126152515411377}, {19.8, 0.0067656636238098145}, {19.85, 0.0066679418087005615}, {19.900000000000002, 0.006978675723075867}, {19.95, 0.006995022296905518}, {20.0, 0.006885826587677002}, {20.05, 0.006692931056022644}, {20.1, 3.5822391510009766e-05}, {20.150000000000002, 2.4527311325073242e-05}]
  out "ms to next point":u32=50500
  in  "Start Fequency":dbl=1.0
  out "Current Sweeping frequency":dbl=0.2
  in  "End Frequency":i32=100
  in  "Frequency Increment":dbl=0.25
  in  "Start Sweep":bool
  out "rail Platform Position":i16=4000
  in  "Half Peirod (pulse 40MHz)":u32=10000
  in  "Rail Desired Position":i16(slide)=4000 scale=0.0..20000.0
  in  "Rail Stepper Direction":bool
  in  "Rail Stepper Enable":bool
  in  "Rail Manual Operation":bool
  in  "LAC Lock":bool
  in  "LAC Position Reset":bool
  in  "LAC Velocity Interval (uSec)":u32=1000
  in  "stop":bool
  in  "VCA Loop Period(us)":i64=2000
  in  "VCA Position Reset":bool
  in  "VCA Velocity Interval (uSec)":u32=1000
  in  "PWM Frequency (default 20kHz)":i32=20000
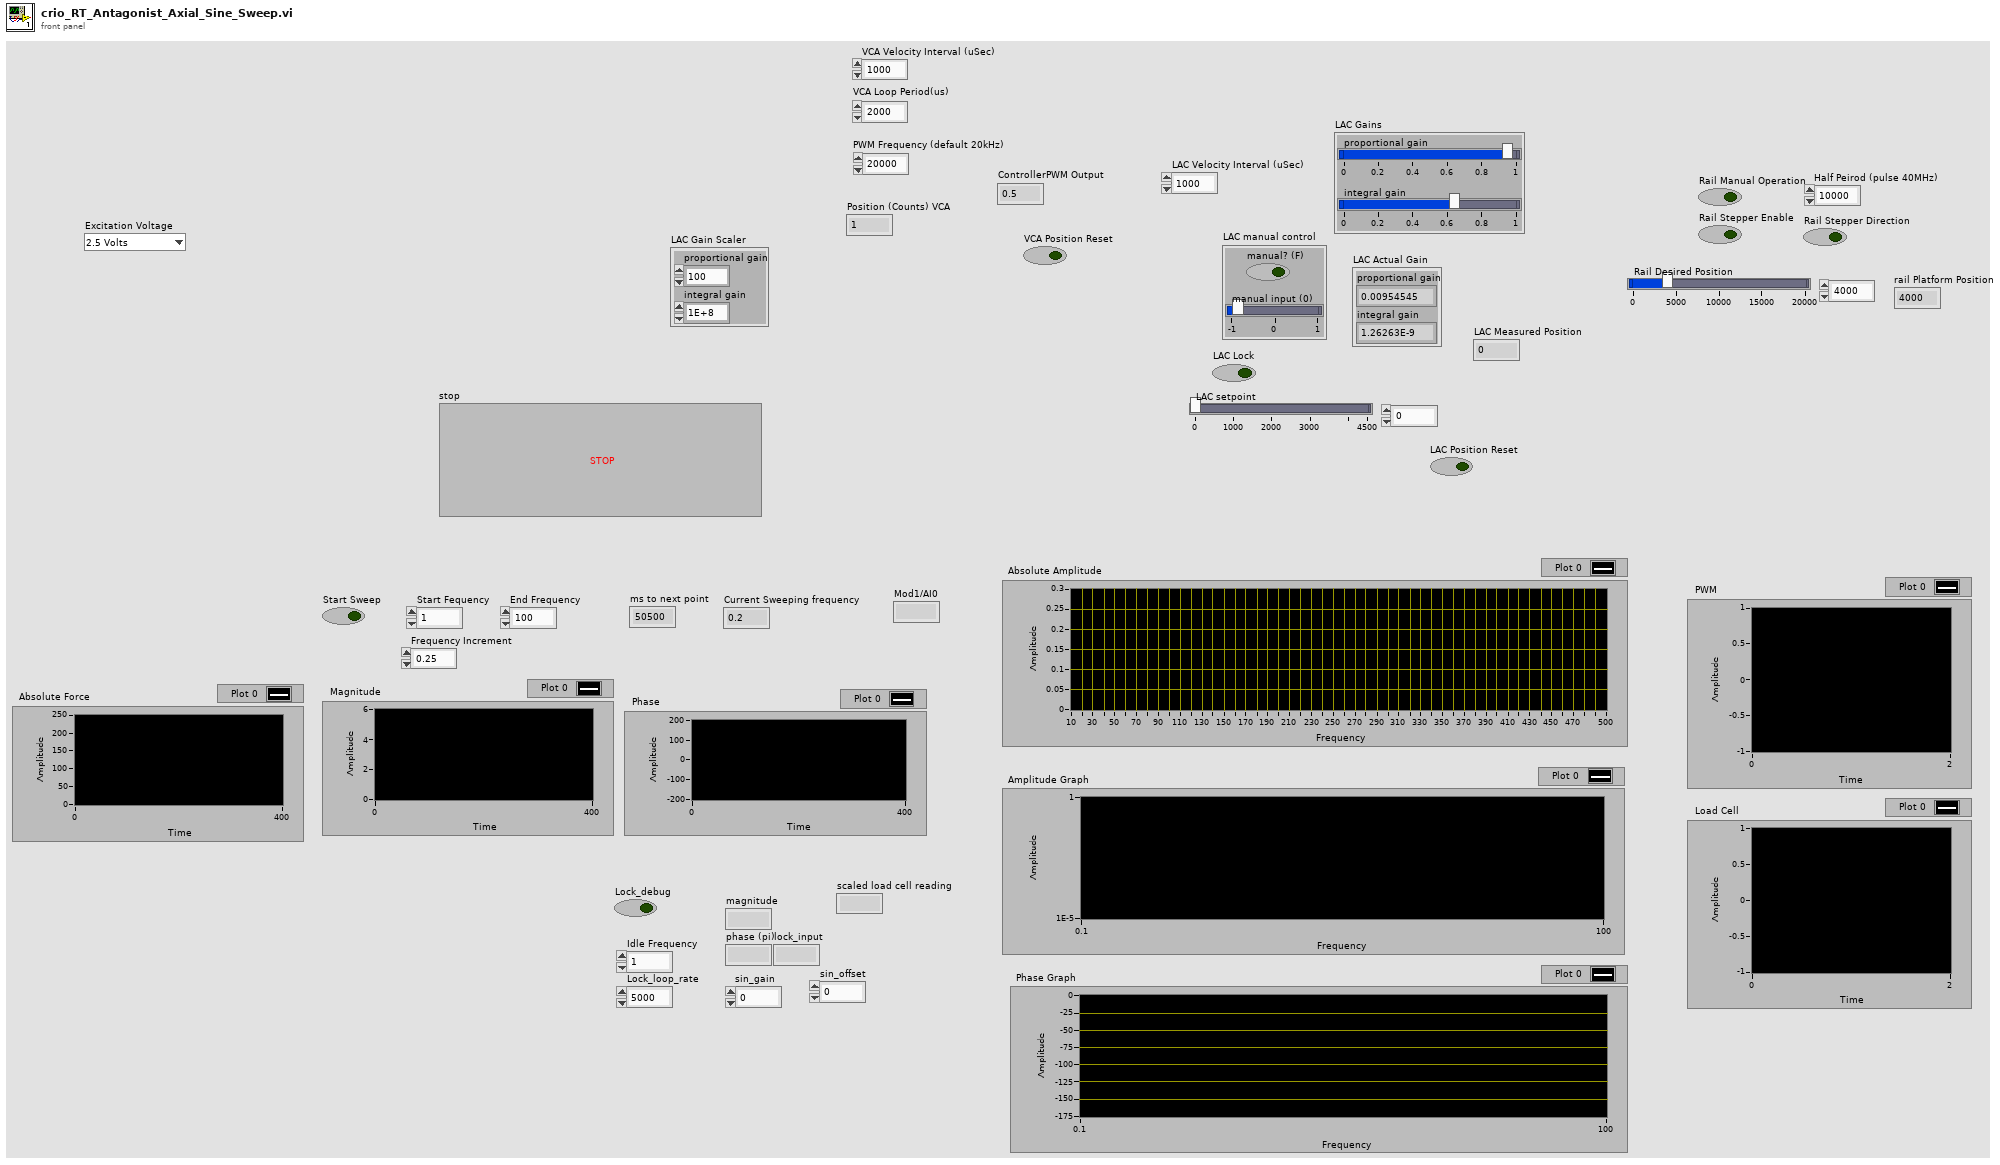
[diagram p1: front panel]
types:
  T1 = cluster{"proportional gain":sgl, "integral gain":sgl}
  T2 = cluster{"manual? (F)":bool, "manual input (0)":sgl}
  T3 = typedef "nicrio_cRIO-9237_ExcitationVoltageRing.ctl" = u8
  T4 = typedef "XDNodeRunTimeDep.lvlib/timing_clust.ctl" = cluster{"Expected End [f-1]":u64, "Actual End [f-1]":u64, "Finished Late? [f-1]":bool, "Expected End [i-1]":u64, "Actual End [i-1]":u64, "Finished Late? [i-1]":bool, "Expected Start [i]":u64, "Actual Start [i]":u64, "Expected Start [f]":u64, "Actual Start [f]":u64, "Source Name":string, "Structure Name":string, "Period":i64, "Deadline":i64, "Offset":i64, "Start":i64, "Priority":i32, "Timeout":i32, "Mode":T5, "Wakeup Reason":T6, "Error":errorcluster, "Source Type":string, "Secondary Source Type":string, "Global End Time":u64, "Global Start Time":u64, "Frame Duration":u64, "Iteration Duration":u64, "Assigned CPU":i32, "I/O Scan Engine Mode":u32}
  T5 = typedef "XDNodeRunTimeDep.lvlib/nitl_modes.ctl" = enum32{"No Change", "Process missed periods, maintain original phase", "Discard missed periods, maintain original phase", "Process missed periods, ignore original phase", "Discard missed periods, ignore original phase"}
  T6 = typedef "XDNodeRunTimeDep.lvlib/wakeup.ctl" = enum32{"Normal", "Aborted", "Asynchronous wakeup", "Timing source error", "Timed loop error", "Timeout"}
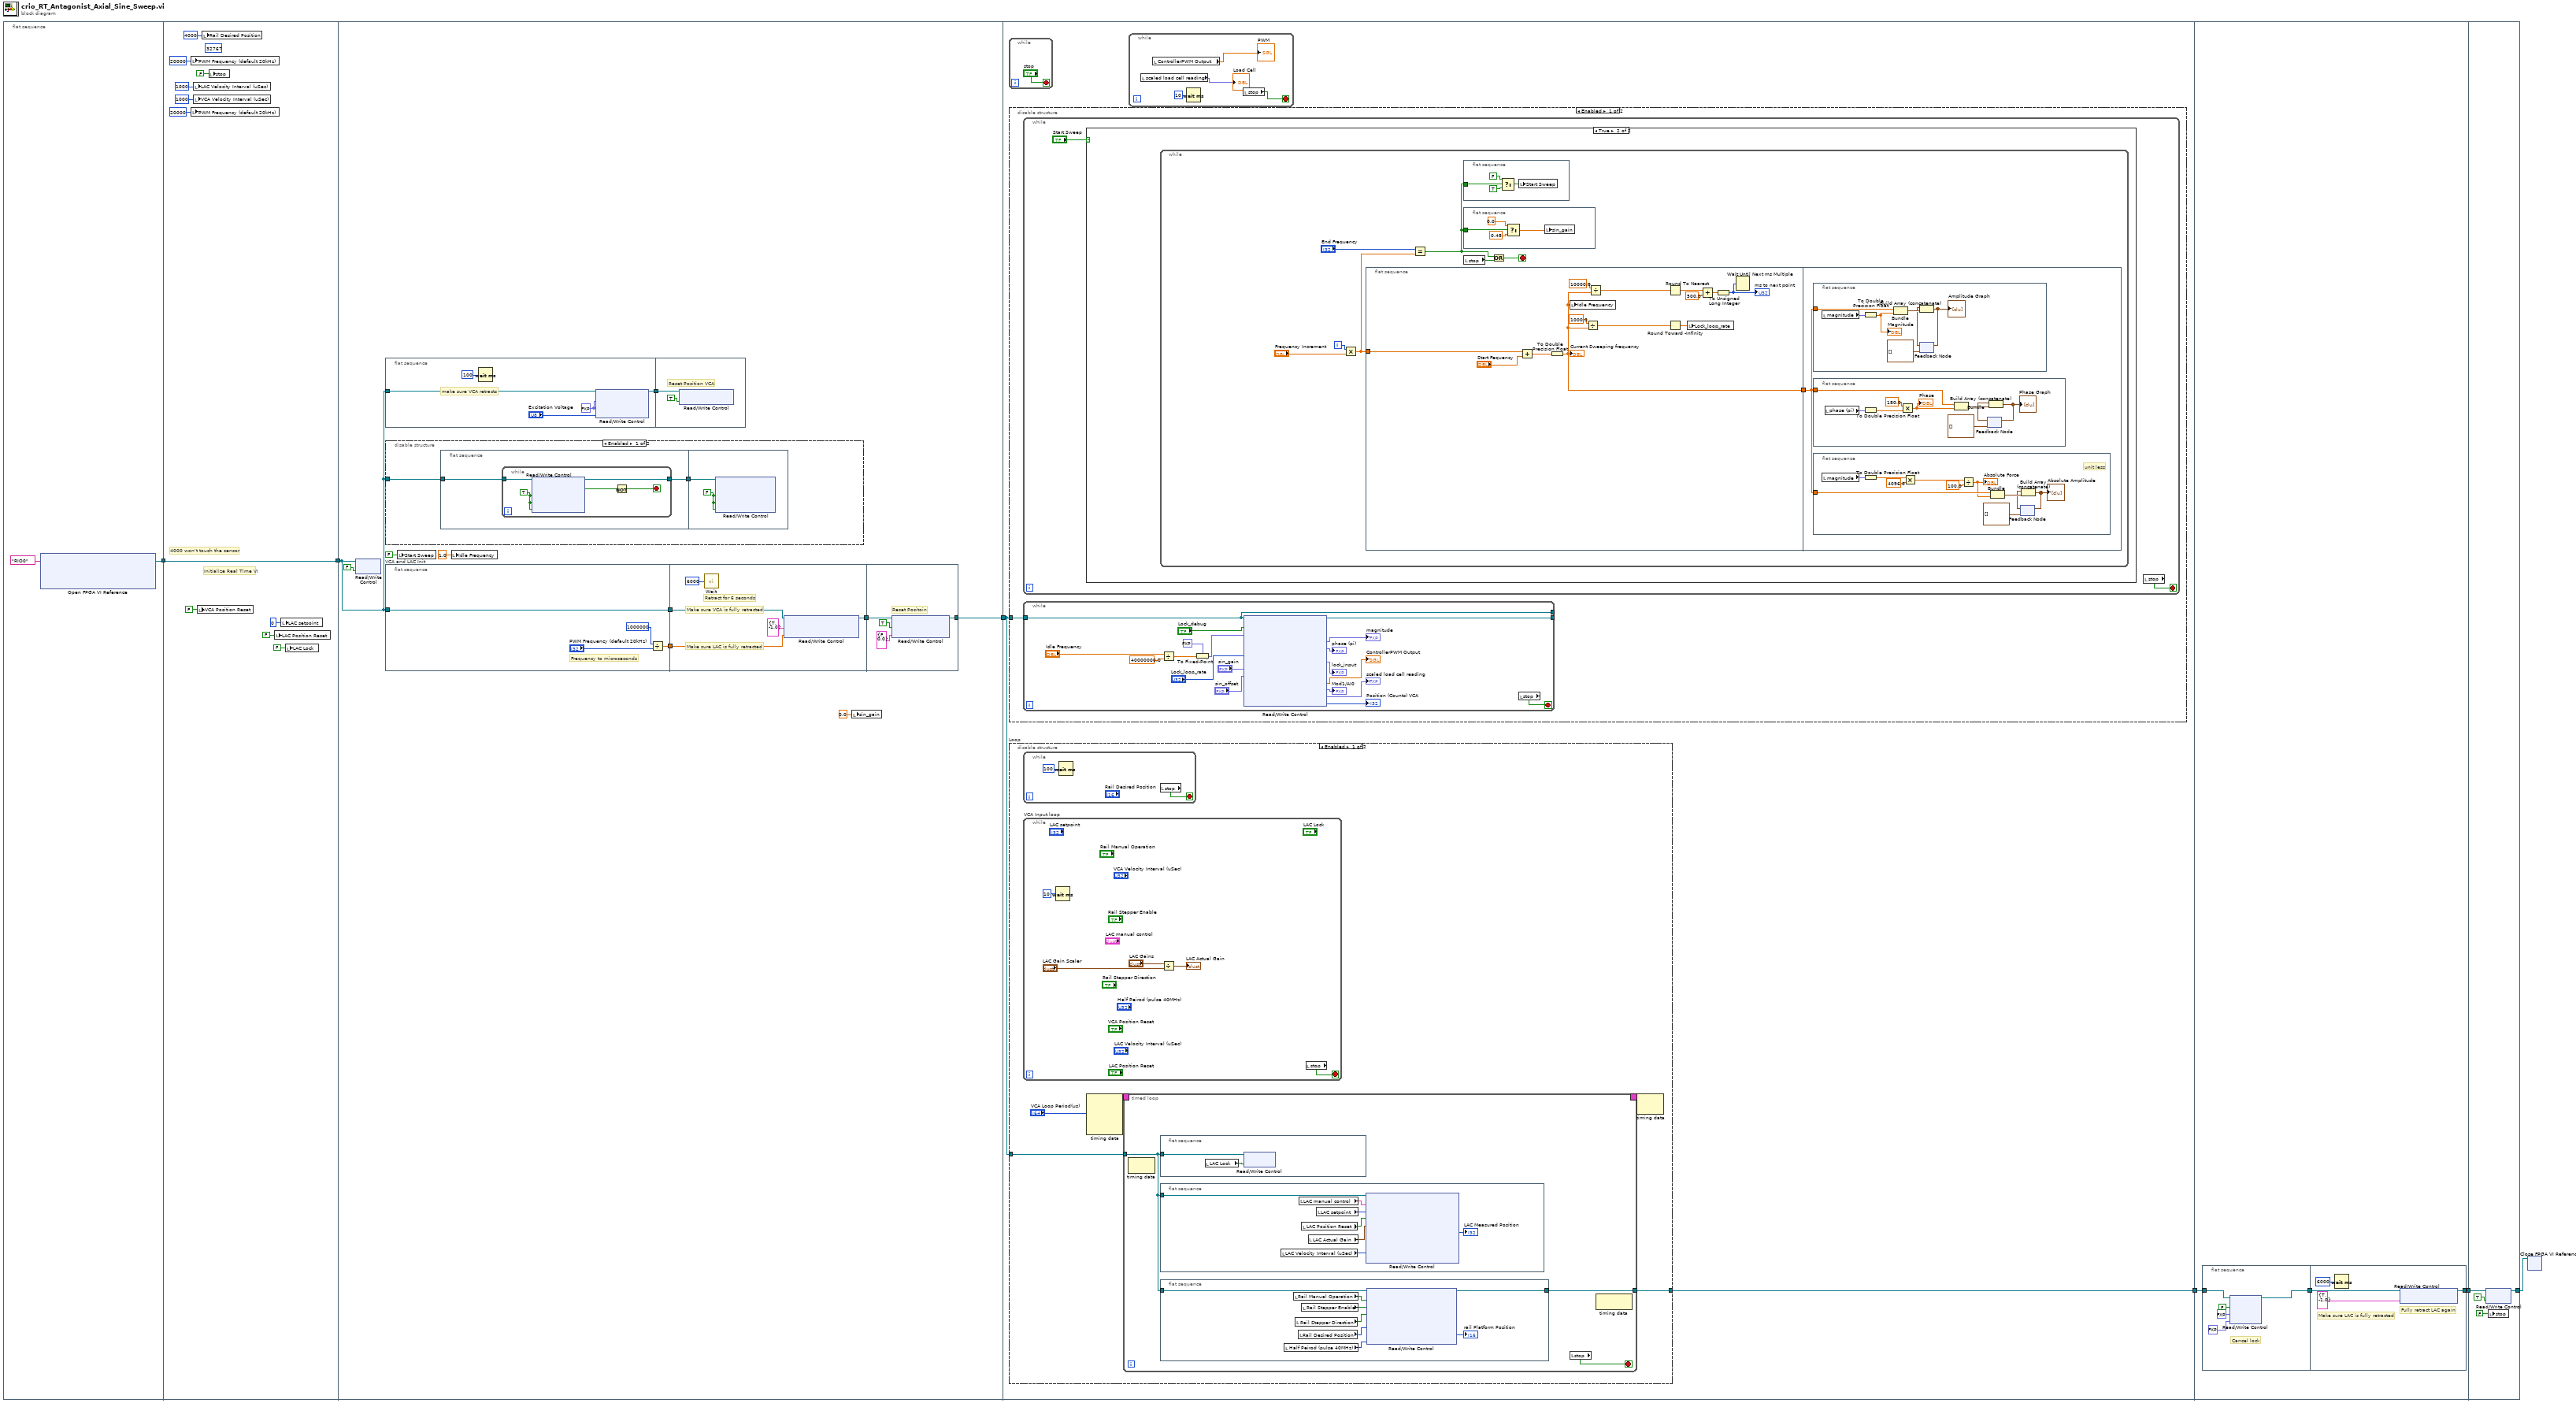
[diagram p0: block diagram]
diagram:
  n1 = flat-sequence {
    tunnel: [w8] -> w1
    tunnel: [w18] -> w6
    tunnel: w1 -> [w18]
    tunnel: [w29] -> w5
    tunnel: w6 -> [w21]
    tunnel: w5 -> [w61]
    tunnel: [w62] -> w3
    tunnel: w3 -> [w187]
    tunnel: [w186] -> w2
    tunnel: w2 -> [w200]
    tunnel: [w199] -> w4
    frame #0 {
      n2 = xnode "Open FPGA VI Reference"("resource name"=tag "RIO0") -> ("FPGA VI Reference Out"=w8:refnum<k20>)  [unwired: 1 in, 1 out]
    }
    frame #1 {
      (unwired) i16 32767 ("Initialize Rail Position")
      # "4000 won't touch the sensor"
      # "Initialize Real Time VI"
      n3 = local write "PWM Frequency (default 20kHz)"(20000 ("PWM Frequency (default 20kHz)")) -> ()
      n4 = local write "PWM Frequency (default 20kHz)"(20000 ("PWM Frequency")) -> ()
      n5 = local write "LAC Velocity Interval (uSec)"(u32 1000 ("Velocity Interval (uSec)")) -> ()
      n6 = local write "VCA Velocity Interval (uSec)"(u32 1000 ("Velocity Interval (uSec)")) -> ()
      n7 = local write "VCA Position Reset"(FALSE ("VCA Position Reset")) -> ()
      n8 = local write "Rail Desired Position"(i16 4000 ("Rail Desired Position")) -> ()
      n9 = local write "stop"(FALSE ("stop")) -> ()
      n10 = local write "LAC Position Reset"(FALSE ("VCA Position Reset")) -> ()
      n11 = local write "LAC setpoint"(0 ("VCA setpoint")) -> ()
      n12 = local write "LAC Lock"(FALSE ("Autolock")) -> ()
    }
    frame #2 {
      n13 = xnode "Read/Write Control"("FPGA VI Reference In"=w21, "stop"=FALSE) -> ()  [unwired: 1 in, 2 out]
      n14 = flat-sequence {
        tunnel: w21 -> [w34]
        tunnel: [w30] -> w20
        tunnel: w20 -> [w35]
        frame #0 {
          w33 = fxp<+/-,16,3> 0.0 ("sin_offset")
          # "make sure VCA retracts"
          n15 = Wait (ms)(milliseconds to wait=u32 100) -> ()  [unwired: 1 out]
          n16 = xnode "Read/Write Control"("FPGA VI Reference In"=w34, "sin_offset"=w33, "sin_gain"=w33, "Excitation Voltage"="Excitation Voltage") -> ("FPGA VI Reference Out"=w30:refnum<k20>)  [unwired: 1 in, 1 out]
        }
        frame #1 {
          # "Reset Position VCA"
          n17 = xnode "Read/Write Control"("FPGA VI Reference In"=w35, "VCA Position Reset"=TRUE ("Position Reset")) -> ()  [unwired: 1 in, 2 out]
        }
      }
      n18 = disable-structure shown="Enabled" {
        disable-tunnel: w21 -> [w37 _]
        frame Enabled {
          n19 = flat-sequence {
            tunnel: w37 -> [w39]
            tunnel: [w40] -> w38
            tunnel: w38 -> [w47]
            frame #0 {
              n20 = while {
                tunnel: [w44] -> w40
                tunnel: w39 -> [w43]
                stop <- w41 stop-if-true
                w45 = TRUE ("Stepper Direction")
                n21 = xnode "Read/Write Control"("FPGA VI Reference In"=w43, "Manual Operation"=w45, "Stepper Enable"=w45, "Stepper Direction"=w45) -> ("FPGA VI Reference Out"=w44:refnum<k20>, "Limit Switch"=w42:bool)  [unwired: 1 in, 1 out]
                n22 = Not(x=w42) -> (.not. x?=w41:bool)
              }
            }
            frame #1 {
              w46 = FALSE ("Stepper Direction")
              n23 = xnode "Read/Write Control"("FPGA VI Reference In"=w47, "Manual Operation"=w46, "Stepper Enable"=w46, "Stepper Direction"=w46) -> ()  [unwired: 1 in, 3 out]
            }
          }
        }
        frame Disabled {
        }
      }
      n24 = flat-sequence "VCA and LAC Init" {
        tunnel: [w50] -> w28
        tunnel: w21 -> [w48]
        tunnel: [w48] -> w27
        tunnel: w28 -> [w55]
        tunnel: w27 -> [w53]
        tunnel: [w56] -> w26
        tunnel: w26 -> [w59]
        tunnel: [w60] -> w29
        frame #0 {
          # "Frequency to microseconds"
          n25 = Divide(x=1000000, y="PWM Frequency (default 20kHz)") -> (x/y=w50:dbl)
        }
        frame #1 {
          # "Make sure LAC is fully retracted"
          # "Retract for 6 seconds"
          # "Make sure VCA is fully retracted"
          n26 = call "Wait"("Count(mSec)"=u32 6000) -> ()  [unwired: 1 out]
          n27 = xnode "Read/Write Control"("FPGA VI Reference In"=w53, "LAC Manual Control"=T2 {"manual? (F)"=TRUE, "manual input (0)"=-1.0} ("manual control"), "DC PWM Period (microsec)"=w55) -> ("FPGA VI Reference Out"=w56:refnum<k20>)  [unwired: 1 in, 1 out]
        }
        frame #2 {
          # "Reset Positoin"
          n28 = xnode "Read/Write Control"("FPGA VI Reference In"=w59, "Position Reset"=TRUE, "LAC Manual Control"=T2 {"manual? (F)"=FALSE, "manual input (0)"=0.0} ("manual control")) -> ("FPGA VI Reference Out"=w60:refnum<k20>)  [unwired: 1 in, 1 out]
        }
      }
      n29 = local write "Start Sweep"(FALSE ("Start Sweep")) -> ()
      n30 = local write "Idle Frequency"(1.0 ("Frequency")) -> ()
      n31 = local write "sin_gain"(0.0 ("Frequency")) -> ()
    }
    frame #3 {
      n32 = while {
        stop <- "stop" stop-if-true
      }
      n33 = disable-structure shown="Enabled" {
        disable-tunnel: w61 -> [w67 _]
        frame Enabled {
          n34 = while {
            stop <- w69 stop-if-true
            n35 = case shown="True" "Start Sweep" {
              frame False {
              }
              frame True {
                n36 = while {
                  i -> [w75]
                  stop <- w77 stop-if-true
                  n37 = Multiply(x=w75, y="Frequency Increment") -> (x*y=w74:dbl)
                  n38 = flat-sequence {
                    tunnel: w74 -> [w91]
                    tunnel: [w86] -> w72
                    tunnel: w72 -> [w99]
                    frame #0 {
                      n39 = Add(x=w91, y="Start Fequency") -> (x+y=w92:dbl)
                      n40 = To Double Precision Float(number=w92) -> (double precision float=w86:dbl)
                      "Current Sweeping frequency" <- w86
                      n41 = local write "Idle Frequency"(w86) -> ()
                      n42 = Divide(x=1000.0 ("y"), y=w86) -> (x/y=w89:dbl)
                      n43 = Divide(x=10000.0 ("y"), y=w86) -> (x/y=w98:dbl)
                      n44 = Round To Nearest(number=w98) -> (nearest integer value=w95:dbl)
                      n45 = Round Toward -Infinity(1:w89) -> (0:w88:dbl)
                      n46 = local write "Lock_loop_rate"(w88) -> ()
                      n47 = Add(x=w95, y=500.0) -> (x+y=w93:dbl)
                      n48 = To Unsigned Long Integer(number=w93) -> (unsigned 32bit integer=w96:u32)
                      "ms to next point" <- w96
                      n49 = Wait Until Next ms Multiple(millisecond multiple=w96) -> ()  [unwired: 1 out]
                    }
                    frame #1 {
                      n50 = flat-sequence {
                        tunnel: w99 -> [w111]
                        frame #0 {
                          n51 = local read "magnitude"() -> (w113:fxp<+,32,6>)
                          n52 = To Double Precision Float(number=w113) -> (double precision float=w112:dbl)
                          "Magnitude" <- w112
                          n53 = Bundle(w111, w112) -> (w117:cluster{dbl, dbl})  [unwired: 1 in]
                          n54 = feedback #1(cluster{dbl, "magnitude":dbl}[] []) -> (w115:cluster{dbl, "magnitude":dbl}[])
                          n55 = Build Array (concatenate)(w115, w117) -> (w114:cluster{dbl, "magnitude":dbl}[])
                          "Amplitude Graph" <- w114
                          n56 = feedback-in #1(w114) -> ()
                        }
                      }
                      n57 = flat-sequence {
                        tunnel: w99 -> [w120]
                        frame #0 {
                          n58 = local read "phase (pi)"() -> (w123:fxp<+/-,16,2>)
                          n59 = To Double Precision Float(number=w123) -> (double precision float=w118:dbl)
                          n60 = Multiply(x=180.0, y=w118) -> (x*y=w119:dbl)
                          "Phase" <- w119
                          n61 = Bundle(w120, w119) -> (w124:cluster{dbl, dbl})  [unwired: 1 in]
                          n62 = feedback #2(cluster{dbl, "magnitude":dbl}[] []) -> (w126:cluster{dbl, "magnitude":dbl}[])
                          n63 = Build Array (concatenate)(w126, w124) -> (w122:cluster{dbl, "magnitude":dbl}[])
                          "Phase Graph" <- w122
                          n64 = feedback-in #2(w122) -> ()
                        }
                      }
                      n65 = flat-sequence {
                        tunnel: w99 -> [w105]
                        frame #0 {
                          # "unit less"
                          n66 = local read "magnitude"() -> (w106:fxp<+,32,6>)
                          n67 = To Double Precision Float(number=w106) -> (double precision float=w104:dbl)
                          n68 = Multiply(x=w104, y=4096.0) -> (x*y=w103:dbl)
                          n69 = Divide(x=w103, y=100.0) -> (x/y=w101:dbl)
                          "Absolute Force" <- w101
                          n70 = Bundle(w105, w101) -> (w110:cluster{dbl, dbl})  [unwired: 1 in]
                          n71 = feedback #3(cluster{dbl, "magnitude":dbl}[] []) -> (w108:cluster{dbl, "magnitude":dbl}[])
                          n72 = Build Array (concatenate)(w108, w110) -> (w107:cluster{dbl, "magnitude":dbl}[])
                          "Absolute Amplitude" <- w107
                          n73 = feedback-in #3(w107) -> ()
                        }
                      }
                    }
                  }
                  n74 = Equal?(x="End Frequency", y=w74) -> (x = y?=w71:bool)
                  n75 = flat-sequence {
                    tunnel: w71 -> [w85]
                    frame #0 {
                      n76 = Select(t=FALSE, s=w85, f=TRUE) -> (s? t:f=w83:bool)
                      n77 = local write "Start Sweep"(w83) -> ()
                    }
                  }
                  n78 = flat-sequence {
                    tunnel: w71 -> [w81]
                    frame #0 {
                      n79 = Select(t=0.0, s=w81, f=0.48) -> (s? t:f=w80:dbl)
                      n80 = local write "sin_gain"(w80) -> ()
                    }
                  }
                  n81 = local read "stop"() -> (w70:bool)
                  n82 = Or(x=w71, y=w70) -> (x .or. y?=w77:bool)
                }
              }
            }
            n83 = local read "stop"() -> (w69:bool)
          }
          n84 = while {
            tunnel: [w128] -> _
            tunnel: [w132] -> _
            tunnel: w67 -> [w128]
            stop <- w145 stop-if-true
            n85 = Divide(x="Idle Frequency", y=40000000.0) -> (x/y=w142:dbl)
            n86 = To Fixed-Point(fixed-point type=fxp<+,32,0> 0.0 ("frequency (periods/tick)"), number=w142) -> (fixed-point=w139:fxp<+,32,0>)
            n87 = xnode "Read/Write Control"("FPGA VI Reference In"=w128, "Lock_debug"="Lock_debug", "sweep frequency (periods/tick)"=w139, "Lock_loop_rate"="Lock_loop_rate", "sin_gain"="sin_gain", "sin_offset"="sin_offset") -> ("FPGA VI Reference Out"=w132:refnum<k20>, "magnitude"=→"magnitude":fxp<+,32,6>, "phase (pi)"=→"phase (pi)":fxp<+/-,16,2>, "lock_input"=→"lock_input":fxp<+/-,24,24>, "ControllerPWM Output"=→"ControllerPWM Output":sgl, "Mod1/AI0"=→"Mod1/AI0":fxp<+/-,24,-4>, "scaled load cell reading"=→"scaled load cell reading":fxp<+/-,24,24>, "Position (Counts) VCA"=→"Position (Counts) VCA":i32)  [unwired: 1 in, 1 out]
            n88 = local read "stop"() -> (w145:bool)
          }
        }
        frame Disabled {
        }
      }
      n89 = disable-structure "Loop" shown="Enabled" {
        disable-tunnel: w61 -> [w147 _]
        disable-tunnel: [w146 _] -> w62
        frame Enabled {
          n90 = while {
            stop <- w151 stop-if-true
            n91 = Wait (ms)(milliseconds to wait=u32 100) -> ()  [unwired: 1 out]
            n92 = local read "stop"() -> (w151:bool)
          }
          n93 = while "VCA Input loop" {
            stop <- w156 stop-if-true
            n94 = Wait (ms)(milliseconds to wait=u32 10) -> ()  [unwired: 1 out]
            n95 = Divide(x="LAC Gains", y="LAC Gain Scaler") -> (x/y=→"LAC Actual Gain":T1)
            n96 = local read "stop"() -> (w156:bool)
          }
          n97 = node-c288("VCA Loop Period(us)") -> (w150:T4)  [unwired: 3 in]
          n98 = timed-loop {
            timing: w150 -> [_]
            timing-out: [_] -> w149
            tunnel: w147 -> [w158]
            tunnel: [w159] -> w146
            stop <- w160 stop-if-true
            n99 = node-c288() -> ()  [unwired: 1 in, 1 out]
            n100 = flat-sequence {
              tunnel: w158 -> [w177]
              frame #0 {
                n101 = local read "LAC Lock"() -> (w176:bool)
                n102 = xnode "Read/Write Control"("FPGA VI Reference In"=w177, "LAC Lock"=w176) -> ()  [unwired: 1 in, 2 out]
              }
            }
            n103 = flat-sequence {
              tunnel: w158 -> [w167]
              frame #0 {
                n104 = local read "LAC Velocity Interval (uSec)"() -> (w162:u32)
                n105 = local read "LAC manual control"() -> (w166:T2)
                n106 = local read "LAC Position Reset"() -> (w164:bool)
                n107 = local read "LAC Actual Gain"() -> (w163:T1)
                n108 = local read "LAC setpoint"() -> (w165:i32)
                n109 = xnode "Read/Write Control"("FPGA VI Reference In"=w167, "LAC Manual Control"=w166, "LAC Setpoint"=w165, "Position Reset"=w164, "LAC Gains"=w163, "LAC Velocity Interval (uSec)"=w162) -> ("LAC Position (Counts)"=→"LAC Measured Position":i32)  [unwired: 1 in, 5 out]
              }
            }
            n110 = flat-sequence {
              tunnel: w158 -> [w169]
              tunnel: [w168] -> w159
              frame #0 {
                n111 = local read "Half Peirod (pulse 40MHz)"() -> (w175:u32)
                n112 = local read "Rail Manual Operation"() -> (w171:bool)
                n113 = local read "Rail Stepper Direction"() -> (w172:bool)
                n114 = local read "Rail Desired Position"() -> (w174:i16)
                n115 = local read "Rail Stepper Enable"() -> (w173:bool)
                n116 = xnode "Read/Write Control"("FPGA VI Reference In"=w169, "Manual Operation"=w171, "Stepper Enable"=w173, "Stepper Direction"=w172, "Position Control: Desired Positoin"=w174, "Half Peirod (pulse 40MHz)"=w175) -> ("FPGA VI Reference Out"=w168:refnum<k20>, "rail Platform Position"=→"rail Platform Position":i16)  [unwired: 2 in, 1 out]
              }
            }
            n117 = local read "stop"() -> (w160:bool)
            n118 = node-c288() -> ()  [unwired: 1 in, 1 out]
          }
          n119 = node-c288(w149) -> ()  [unwired: 1 out]
        }
        frame Disabled {
        }
      }
      n120 = while {
        stop <- w65 stop-if-true
        n121 = local read "scaled load cell reading"() -> (→"Load Cell":fxp<+/-,24,24>)
        n122 = local read "ControllerPWM Output"() -> (→"PWM":sgl)
        n123 = Wait (ms)(milliseconds to wait=u32 10) -> ()  [unwired: 1 out]
        n124 = local read "stop"() -> (w65:bool)
      }
    }
    frame #4 {
      n125 = flat-sequence {
        tunnel: w187 -> [w192]
        tunnel: [w191] -> w185
        tunnel: [w195] -> w186
        tunnel: w185 -> [w196]
        frame #0 {
          # "Cancel lock"
          n126 = xnode "Read/Write Control"("FPGA VI Reference In"=w192, "LAC Lock"=FALSE, "sin_offset"=fxp<+/-,16,3> -1.0, "sin_gain"=fxp<+,32,1> 0.0) -> ("FPGA VI Reference Out"=w191:refnum<k20>)  [unwired: 1 in, 1 out]
        }
        frame #1 {
          # "Make sure LAC is fully retracted"
          # "Fully retract LAC again"
          n127 = Wait (ms)(milliseconds to wait=u32 6000) -> ()  [unwired: 1 out]
          n128 = xnode "Read/Write Control"("FPGA VI Reference In"=w196, "LAC Manual Control"=T2 {"manual? (F)"=TRUE, "manual input (0)"=-1.0} ("manual control")) -> ("FPGA VI Reference Out"=w195:refnum<k20>)  [unwired: 1 in, 1 out]
        }
      }
    }
    frame #5 {
      n129 = xnode "Read/Write Control"("FPGA VI Reference In"=w200, "stop"=TRUE) -> ("FPGA VI Reference Out"=w199:refnum<k20>)  [unwired: 1 in, 1 out]
      n130 = local write "stop"(FALSE ("stop")) -> ()
    }
  }
  n131 = xnode "Close FPGA VI Reference"("FPGA VI Reference In"=w4) -> ()  [unwired: 1 in, 1 out]
